vi "t3_parse_stream_v2.vi"(6 "first_batch?":bool, 7 "Last_sync":cluster{"sync_counter":i32, "sync_time":i64}, 8 "Error In":errorcluster, 9 "stamps":i64[](array[numeric]), 10 "channels":u32[](array[numeric]), 11 "reference_channel":i32) -> (0 "Error In 2":errorcluster, 1 "count_timestamps":i64[](array[numeric]), 2 "n_sync array":i32[](array[numeric]), 3 "channels":u32[](array[numeric]), 4 "first_batch?":bool, 5 "last_sync_out":cluster{"sync_counter":i32, "sync_time":i64})   [LabVIEW 2018]
panel:
  out "output variable 2":u64[](array[numeric])
  out "output variable":i32[](array[numeric])
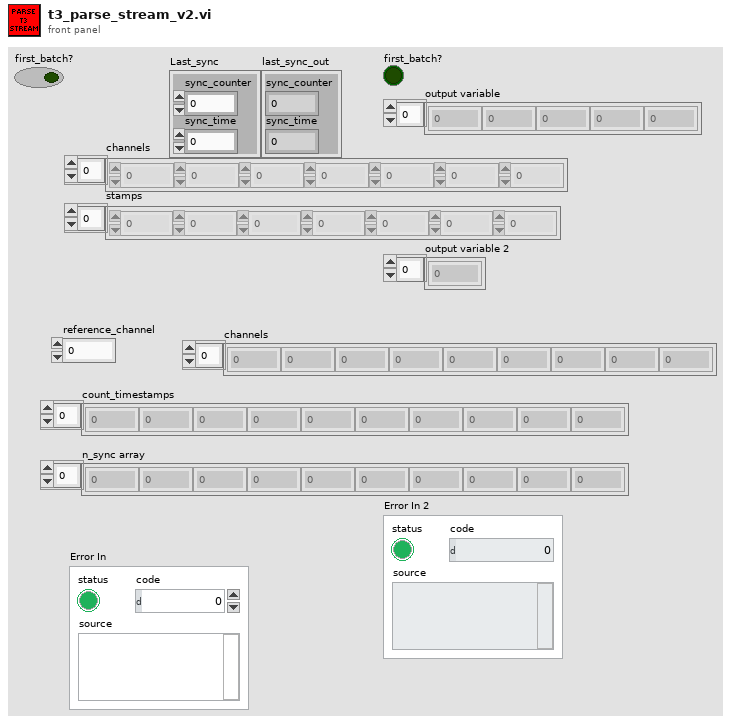
[diagram p1: front panel]
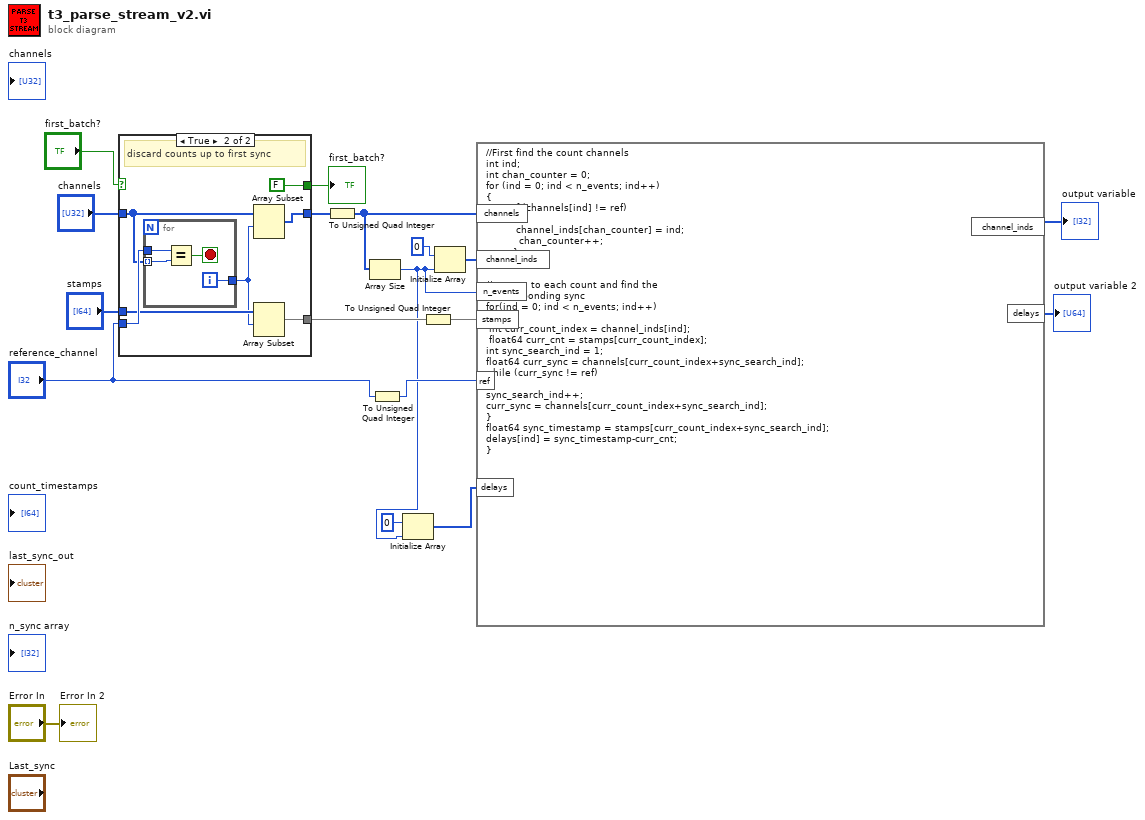
[diagram p0: block diagram]
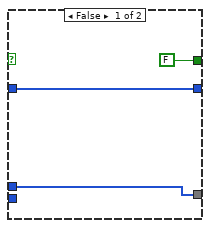
[diagram p2: hidden frame]
diagram:
  n1 = case shown="True" "first_batch?" {
    tunnel: "reference_channel" -> [_ w28]
    tunnel: "channels" -> [w21 w27]
    tunnel: [w21 w26] -> w12
    tunnel: "stamps" -> [w20 w25]
    tunnel: [w20 w23] -> w13
    tunnel: [FALSE FALSE] -> w14
    frame False {
    }
    frame True {
      # "discard counts up to first sync"
      n2 = for {
        tunnel: w28 -> [w31]
        tunnel: w27 -> [w32] mode=indexing
        tunnel: [w30] -> w24
        i -> [w30]
        stop <- w29 stop-if-true
        n3 = Equal?(x=w31, y=w32) -> (x = y?=w29:bool)
      }
      n4 = Array Subset(array=w27, index=w24) -> (w26:u32[])  [unwired: 1 in]
      n5 = Array Subset(array=w25, index=w24) -> (w23:i64[])  [unwired: 1 in]
    }
  }
  "first_batch?" <- w14
  n6 = To Unsigned Quad Integer(1:w12) -> (0:w10:u64[])
  n7 = Array Size(array=w10) -> (size(s)=w2:i32)
  n8 = To Unsigned Quad Integer(1:"reference_channel") -> (0:w5:u64)
  n9 = Initialize Array(u64 0 ("element"), w2) -> (w4:u64[])
  n10 = To Unsigned Quad Integer(1:w13) -> (0:w11:u64[])
  n11 = Initialize Array(0 ("element"), w2) -> (w8:i32[])
  n12 = formula code="//First find the count channels\nint ind;\nint chan_counter = 0;\nfor (ind = 0; ind < n_events; ind++)\n{\n         if (channels[ind] != ref)\n         {\n          channel_inds[chan_counter] = ind;\n           chan_counter++;\n         }\n}\n\n//next go to each count and find the\n//corresponding sync\nfor(ind = 0; ind < n_events; ind++)\n{\n int curr_count_index = channel_inds[ind];\n float64 curr_cnt = stamps[curr_count_index];\nint sync_search_ind = 1;\nfloat64 curr_sync = channels[curr_count_index+sync_search_ind];\nwhile (curr_sync != ref)\n{\nsync_search_ind++;\ncurr_sync = channels[curr_count_index+sync_search_ind];\n}\nfloat64 sync_timestamp = stamps[curr_count_index+sync_search_ind];\ndelays[ind] = sync_timestamp-curr_cnt;\n}"("channels"=w10, "stamps"=w11, "ref"=w5, "channel_inds"=w8, "n_events"=w2, "delays"=w4) -> ("channel_inds"=→"output variable":i32[], "delays"=→"output variable 2":u64[])
  "Error In 2" <- "Error In"
